vi "uintDivide.vi"(8 "Error in (no error)":errorcluster, 10 "Uint2 in":refnum<class "UintClass.lvclass">, 11 "Uint1 in":refnum<class "UintClass.lvclass">) -> (0 "Error out":errorcluster, 1 "Timing":u32, 2 "floor(Uint1/Uint2)":refnum<class "UintClass.lvclass">, 3 "Uint1 mod Uint2":refnum<class "UintClass.lvclass">, 5 "Timeout?":bool)   [LabVIEW 2011, in "UintClass.lvclass"]
uses:
  UintClass.lvclass
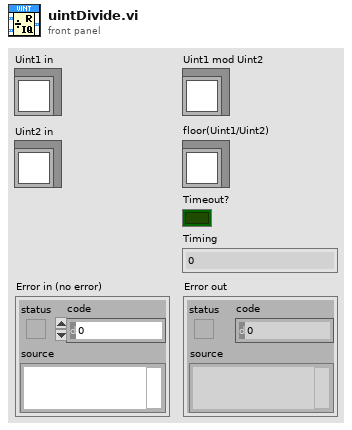
[diagram p1: front panel]
types:
  T1 = typedef "UintClass.lvclass/timeout.ctl" = i32
  T2 = typedef "UintClass.lvclass/enumBase.ctl" = u16
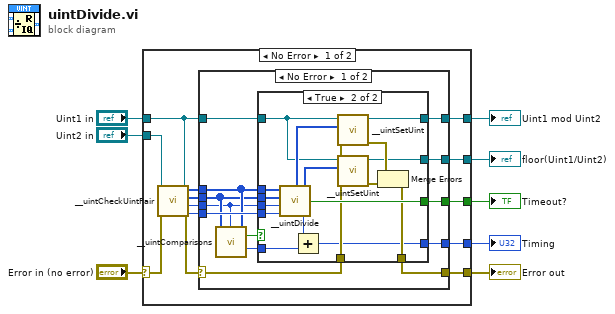
[diagram p0: block diagram]
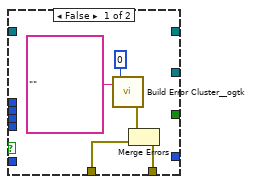
[diagram p2: hidden frame]
diagram:
  n1 = case shown="No Error" "Error in (no error)" {
    selector: "Error in (no error)" -> [w18 w58]
    tunnel: [w16 w58] -> w7
    tunnel: "Uint2 in" -> [w19 _]
    tunnel: "Uint1 in" -> [w11 _]
    tunnel: [w21 _] -> w4
    tunnel: [w20 _] -> w3
    tunnel: [w10 _] -> w2
    tunnel: [w9 _] -> w1
    frame No Error {
      n2 = call "__uintCheckUintPair.vi"("Error in (no error)"=w18, "Uint2 in"=w19, "Uint1 in"=w11) -> ("Error out"=w17:errorcluster, "Timeout (-1)"=w13:T1, "Uint2 out"=w14:u8[], "Uint1 out"=w15:u8[], "Base out"=w12:T2)  [unwired: 4 in]
      n3 = case shown="No Error" w17 {
        selector: w17 -> [w30 w57]
        tunnel: [w34 _] -> w21
        tunnel: [w33 _] -> w20
        tunnel: [w29 w57] -> w16
        tunnel: w15 -> [w27 _]
        tunnel: w14 -> [w26 _]
        tunnel: w13 -> [w23 _]
        tunnel: w12 -> [w32 _]
        tunnel: w11 -> [w31 _]
        tunnel: [w28 _] -> w10
        tunnel: [w25 _] -> w9
        frame No Error {
          n4 = call "__uintComparisons.vi"("Timeout (-1)"=w23, "Uint2 in"=w26, "Uint1 in"=w27) -> ("Timing comparison"=w22:u32, "Uint1 > Uint2"=w24:bool)  [unwired: 1 in, 6 out]
          n5 = case shown="True" w24 {
            tunnel: [_ w42] -> w34
            tunnel: [_ w55] -> w33
            tunnel: w23 -> [_ w54]
            tunnel: w32 -> [_ w53]
            tunnel: w31 -> [_ w45]
            tunnel: w30 -> [w39 w49]
            tunnel: [w38 w46] -> w29
            tunnel: [_ w52] -> w28
            tunnel: w27 -> [_ w51]
            tunnel: w26 -> [_ w50]
            tunnel: [_ w43] -> w25
            tunnel: w22 -> [_ w40]
            frame False {
              n6 = call <userlib>:"Build Error Cluster__ogtk.vi"("String to Prepend to source (\"\")"="" ("String to Prepend to source (\"\")"), "code"=0) -> ("error out"=w37:errorcluster)
              n7 = Merge Errors(w37, w39) -> (w38:errorcluster)
            }
            frame True {
              n8 = call "__uintDivide.vi"("Base (decimal)"=w53, "Timeout (-1)"=w54, "Uint2 in"=w50, "Uint1 in"=w51) -> ("Timing division"=w41:u32, "Timeout?"=w52:bool, "floor(Uint1 / Uint1)"=w44:u8[], "Uint1 mod Uint2"=w56:u8[])
              n9 = Add(x=w41, y=w40) -> (x+y=w42:u32)
              n10 = call "__uintSetUint.vi"("Error in (no error)"=w49, 10:"Uint in"=w56, 11:"Uint in"=w45) -> ("Error out"=w48:errorcluster, "Uint out"=w55:refnum<class "UintClass.lvclass">)  [unwired: 7 in]
              n11 = call "__uintSetUint.vi"("Error in (no error)"=w49, 10:"Uint in"=w44, 11:"Uint in"=w45) -> ("Error out"=w47:errorcluster, "Uint out"=w43:refnum<class "UintClass.lvclass">)  [unwired: 7 in]
              n12 = Merge Errors(w48, w47) -> (w46:errorcluster)
            }
          }
        }
        frame Error {
        }
      }
    }
    frame Error {
    }
  }
  "Error out" <- w7
  "Uint1 mod Uint2" <- w3
  "Timing" <- w4
  "Timeout?" <- w2
  "floor(Uint1/Uint2)" <- w1
